vi "Pre-Install Custom Action.vi"(10 "Variant":variant) -> (0 "error out":errorcluster)   [LabVIEW 2020]
uses:
  <vilib>/OpenLvVision/OpenLvVision_OpenCv/Installer/ControlRefs.ctl
  <vilib>/OpenLvVision/OpenLvVision_OpenCv/Installer/FileElement.ctl
panel:
  out "SubTask_Slider":dbl(slide) scale=0.0..1.1025
  out "MainTask_Slider":dbl(slide) scale=0.0..6.0
  in  "Offline":bool
  in  "Cancel":bool
  out "SubTask_Text":string
  out "MainTask_Text":string="Installer Started"
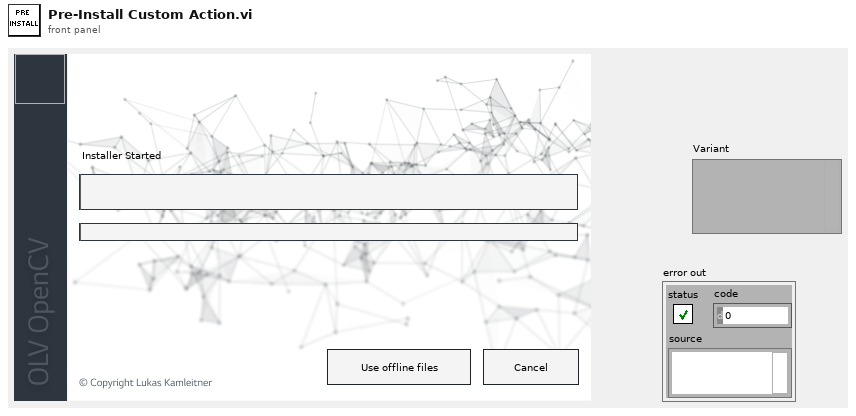
[diagram p1: front panel]
types:
  T1 = typedef "OLV_InstallerOpenCV.lvlib/ControlRefs.ctl" = cluster{"MainTask_Slider":refnum<vi>, "SubTask_Slider":refnum<vi>, "MainTask_Text":refnum<vi>, "SubTask_Text":refnum<vi>, "Offline":refnum<vi>, "Cancel":refnum<vi>}
  T2 = enum32{"Invalid", "Standard", "Closed", "Hidden", "Minimized", "Maximized"}
  T3 = typedef "OLV_InstallerOpenCV.lvlib/FileElement.ctl" = cluster{"Url":string, "ByteSize":i64}
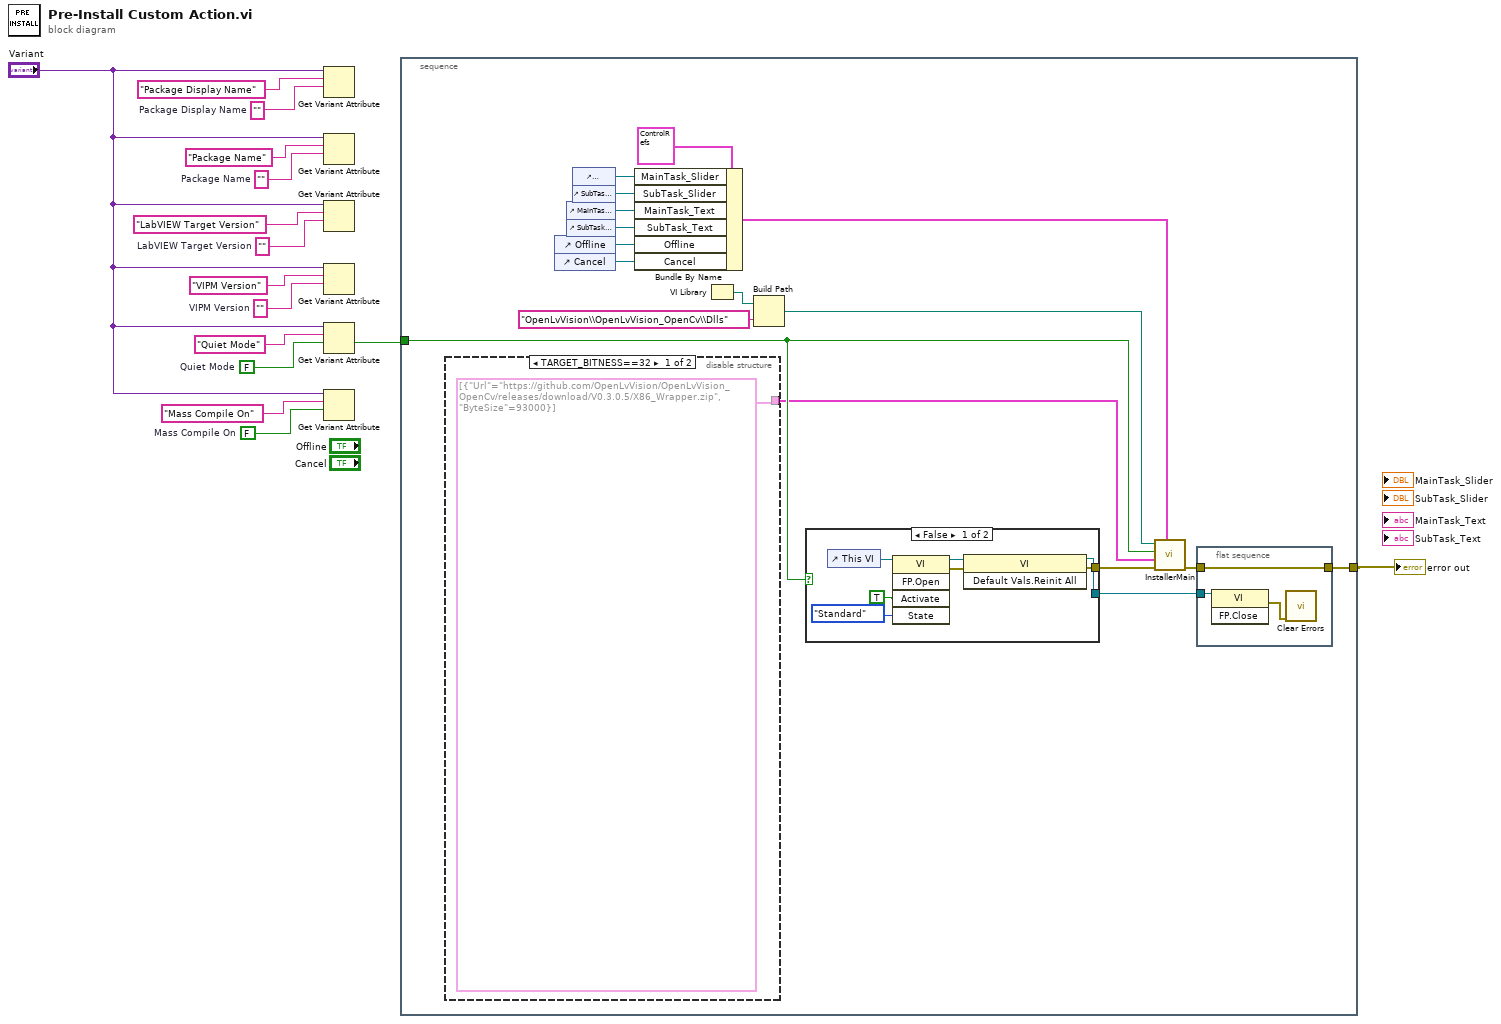
[diagram p0: block diagram]
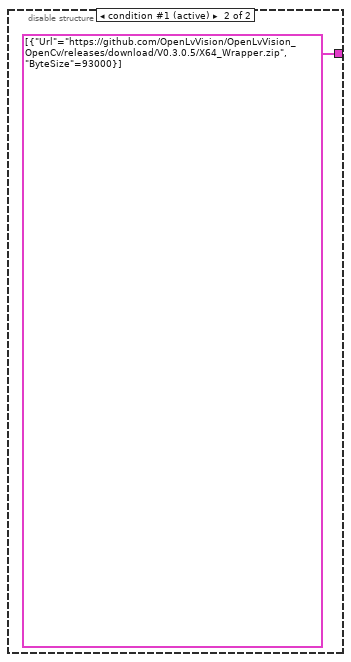
[diagram p3: hidden frame]
diagram:
  w3 = FALSE  # Mass Compile On
  w5 = ""  # Package Display Name
  w6 = FALSE  # Quiet Mode
  w9 = ""  # VIPM Version
  w11 = ""  # LabVIEW Target Version
  w13 = ""  # Package Name
  n1 = Get Variant Attribute(Variant="Variant", name="Package Display Name", default value (empty Variant)=w5) -> ()  [unwired: 1 in, 4 out]
  n2 = Get Variant Attribute(Variant="Variant", name="Package Name", default value (empty Variant)=w13) -> ()  [unwired: 1 in, 4 out]
  n3 = Get Variant Attribute(Variant="Variant", name="LabVIEW Target Version", default value (empty Variant)=w11) -> ()  [unwired: 1 in, 4 out]
  n4 = Get Variant Attribute(Variant="Variant", name="VIPM Version", default value (empty Variant)=w9) -> ()  [unwired: 1 in, 4 out]
  n5 = Get Variant Attribute(Variant="Variant", name="Quiet Mode", default value (empty Variant)=w6) -> (value=w2:bool)  [unwired: 1 in, 3 out]
  n6 = Get Variant Attribute(Variant="Variant", name="Mass Compile On", default value (empty Variant)=w3) -> ()  [unwired: 1 in, 4 out]
  n7 = stacked-sequence {
    tunnel: w2 -> [w17]
    tunnel: [w19] -> w1
    frame #0 {
      n8 = disable-structure shown="TARGET_BITNESS==32" {
        disable-tunnel: [T3[] [{"Url"="https://github.com/OpenLvVision/OpenLvVision_OpenCv/releases/download/V0.3.0.5/X86_Wrapper.zip", "ByteSize"=93000}] T3[] [{"Url"="https://github.com/OpenLvVision/OpenLvVision_OpenCv/releases/download/V0.3.0.5/X64_Wrapper.zip", "ByteSize"=93000}]] -> w16
        frame condition #0 {
        }
        frame condition #1 (active) {
        }
      }
      n9 = control-ref of="Offline"() -> (w24:refnum<vi>)
      n10 = control-ref of="Cancel"() -> (w23:refnum<vi>)
      n11 = control-ref of="MainTask_Text"() -> (w26:refnum<vi>)
      n12 = control-ref of="SubTask_Text"() -> (w25:refnum<vi>)
      n13 = control-ref of="MainTask_Slider"() -> (w28:refnum<vi>)
      n14 = control-ref of="SubTask_Slider"() -> (w27:refnum<vi>)
      n15 = Bundle By Name(cluster=T1 {"MainTask_Slider"=refnum, "SubTask_Slider"=refnum, "MainTask_Text"=refnum, "SubTask_Text"=refnum, "Offline"=refnum, "Cancel"=refnum} ("CtlRefs"), "MainTask_Slider"=w28, "SubTask_Slider"=w27, "MainTask_Text"=w26, "SubTask_Text"=w25, "Offline"=w24, "Cancel"=w23) -> (w22:T1)
      n16 = VI Library() -> (path=w32:path)
      n17 = Build Path(base path=w32, name or relative path="OpenLvVision\\OpenLvVision_OpenCv\\Dlls") -> (appended path=w30:path)
      n18 = case shown="False" w17 {
        tunnel: [w34 _] -> w21
        tunnel: [w33 _] -> w18
        frame False {
          n19 = control-ref of="This VI"() -> (w35:refnum<vi>)
          n20 = invoke class="VI" method="FP.Open"(reference=w35, "Activate"=TRUE ("Activate?"), "State"=T2."Standard") -> (reference out=w37:refnum<vi>, error out=w36:errorcluster)  [unwired: 2 in, 3 out]
          n21 = invoke class="VI" method="Default Vals.Reinit All"(reference=w37, error in=w36) -> (reference out=w33:refnum<vi>, error out=w34:errorcluster)  [unwired: 1 in, 1 out]
        }
        frame True {
        }
      }
      n22 = call <vilib>:"InstallerMain.vi"("CtlRefs"=w22, "error in"=w21, "Files"=w16, "Quiet"=w17, "InstallFolderPath"=w30) -> ("error out"=w20:errorcluster)  [unwired: 6 in]
      n23 = flat-sequence {
        tunnel: w20 -> [w42]
        tunnel: [w42] -> w19
        tunnel: w18 -> [w41]
        frame #0 {
          n24 = invoke class="VI" method="FP.Close"(reference=w41) -> (error out=w40:errorcluster)  [unwired: 2 in, 2 out]
          n25 = call <vilib>:"Clear Errors.vi"("error in (no error)"=w40) -> ()  [unwired: 5 in, 2 out]
        }
      }
    }
  }
  "error out" <- w1
